vi "Finding-g.vi"() -> ()   [LabVIEW 2021]
uses:
  <userlib>/ImageProcessing/IdentifyBlob_Circle_Cluster.vi
  _SubVis/Ramp.vi
  _SubVis/Bounce.vi
panel:
  out "Cropped Data":dbl[](graph)
  out "Image 3":picture
  in  "stop":bool
  in  "Bounce":bool
  in  "Ramp":bool
  out "Acceleration due to gravity =":dbl
  out "Distance Chart":dbl[](graph)
  # "m/s/s"
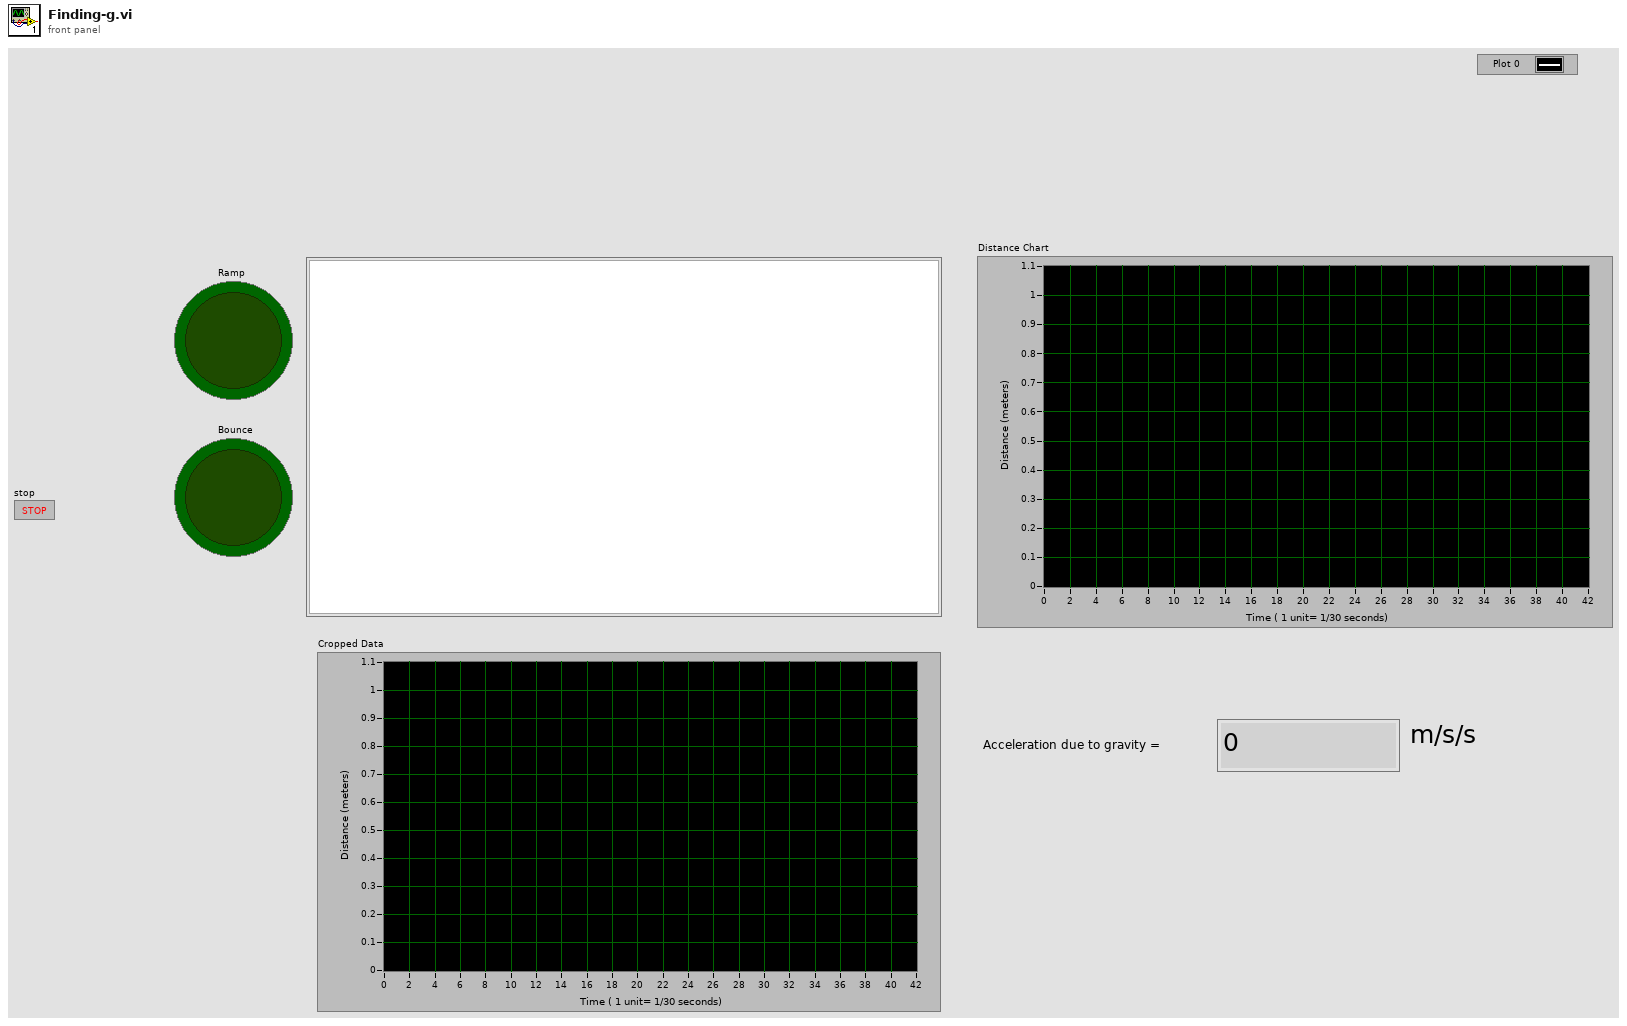
[diagram p1: front panel]
types:
  T1 = typedef "QT_Image.ctl" = cluster{"Width":i32, "Height":i32, "Depth":i32, "data":u8[], "Compressed data":u8[], "Color table":u32[], "Duration":i32, "Options":i32, "Timestamp":i32, "ID":i32, "Reserved":i32, "Dialogs":u32}
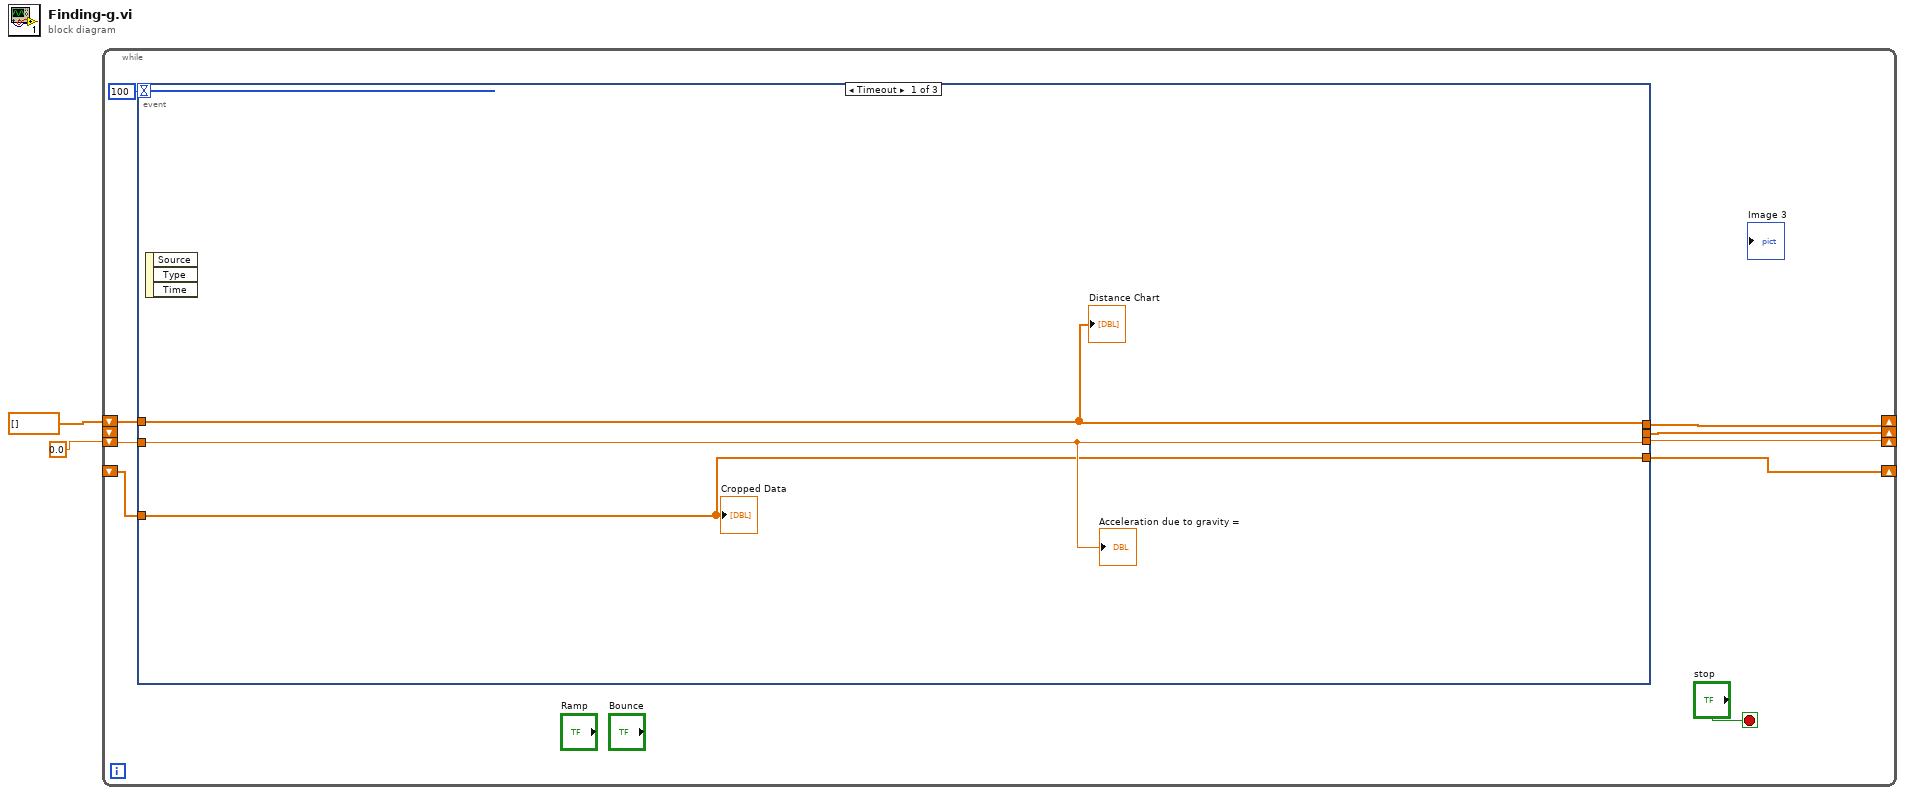
[diagram p0: block diagram]
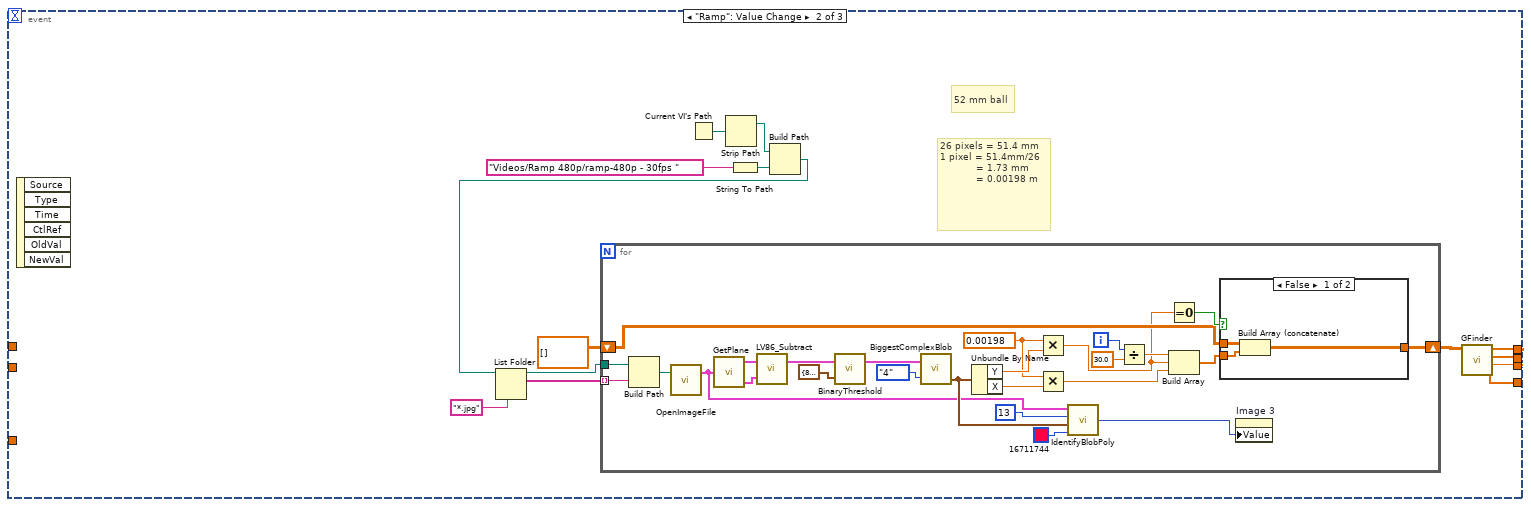
[diagram p2: hidden frame]
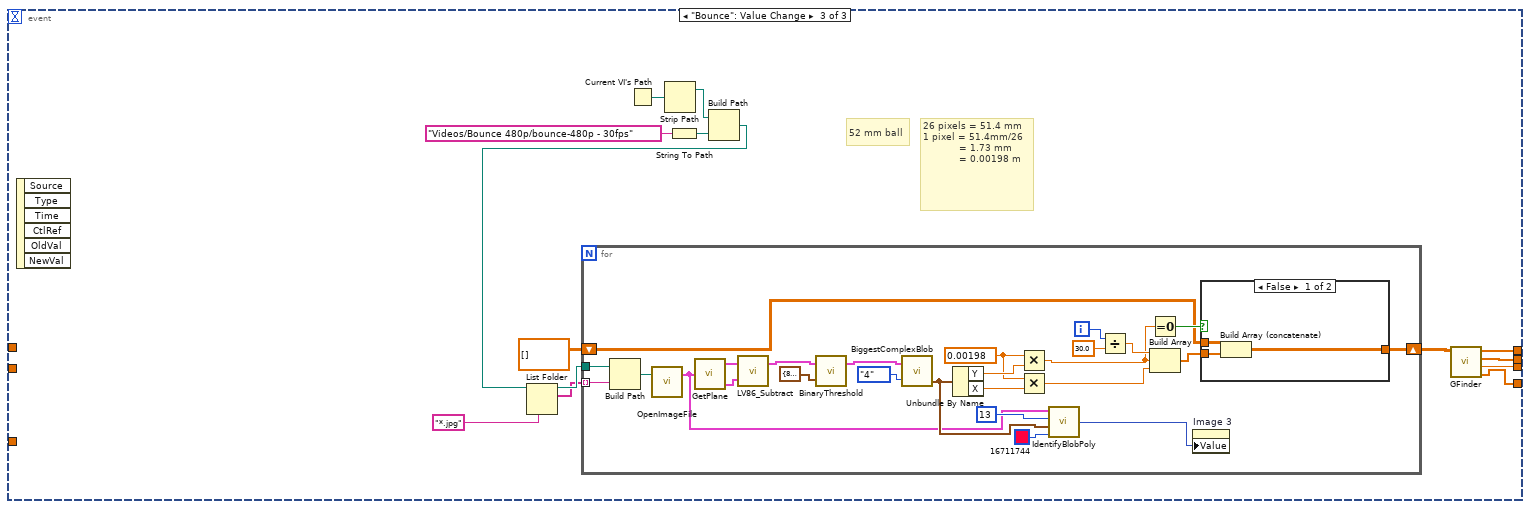
[diagram p4: hidden frame]
diagram:
  n1 = while {
    shift-right: [w7] -> _
    shift-left: dbl[] [] ("Distance") -> [w9]
    shift-right: [w6] -> _
    shift-left: 0.0 ("Acceleration") -> [w8]
    shift-right: [w5] -> _
    shift-left: _ -> [w3]
    shift-right: [w4] -> _
    shift-left: _ -> [_]
    stop <- "stop" stop-if-true
    n2 = event shown="[0] Timeout" {
      selector: _ -> [_ _ _]
      dyn-events: _ -> [_ _ _]
      timeout: 100 -> [_ _ _]
      tunnel: [w14 w22 w71] -> w6
      tunnel: [w13 w23 w72] -> w7
      tunnel: w9 -> [w13 _ _]
      tunnel: w8 -> [w14 _ _]
      tunnel: [w12 w21 w65] -> w5
      tunnel: [_ w20 w64] -> w4
      tunnel: w3 -> [w12 _ _]
      event Timeout {
        n3 = event-data() -> ()  [unwired: 1 in, 3 out]
        "Distance Chart" <- w13
        "Acceleration due to gravity =" <- w14
        "Cropped Data" <- w12
      }
      event "Ramp": Value Change {
        # "26 pixels = 51.4 mm\n1 pixel = 51.4mm/26\n            = 1.73 mm\n            = 0.00198 m"
        # "52 mm ball"
        n4 = event-data() -> ()  [unwired: 1 in, 6 out]
        n5 = Current VI's Path() -> (path=w19:path)
        n6 = Strip Path(path=w19) -> (stripped path=w18:path)  [unwired: 1 out]
        n7 = String To Path(string="Videos/Ramp 480p/ramp-480p - 30fps ") -> (path=w16:path)
        n8 = Build Path(base path=w18, name or relative path=w16) -> (appended path=w15:path)
        n9 = List Folder(path=w15, pattern="*.jpg" ("string")) -> (path out=w27:path, filenames=w26:string[])  [unwired: 2 in, 2 out]
        n10 = for {
          tunnel: w26 -> [w53] mode=indexing
          tunnel: w27 -> [w54]
          shift-right: [w44] -> w24
          shift-left: dbl[][] [] -> [w46]
          i -> [w42]
          w34 = 0.00198 ("x")
          n11 = Build Path(base path=w54, name or relative path=w53) -> (appended path=w52:path)
          n12 = call <userlib>:"OpenImageFile.vi"("selected path"=w52) -> ("Image Out"=w40:T1)  [unwired: 2 in]
          n13 = call <userlib>:"GetPlane.vi"("Image In"=w40) -> ("Blue Plane Out"=w39:T1, "Red Plane Out"=w38:T1)  [unwired: 1 out]
          n14 = call <userlib>:"LV86_Subtract.vi"("Image 2"=w39, "Image"=w38) -> ("Image Out"=w37:T1)  [unwired: 1 in]
          n15 = call <userlib>:"BinaryThreshold.vi"("threshold"=cluster{u8, u8} {82, 120} ("Red Threshold"), "Image In"=w37) -> ("Image Out"=w36:T1)  [unwired: 1 in]
          n16 = call <userlib>:"BiggestComplexBlob.vi"("Connectivity"=enum16{"4", "8"}."4", "Image in"=w36) -> ("Centroid"=w51:cluster{"X":dbl, "Y":dbl})  [unwired: 2 out]
          n17 = Unbundle By Name(w51) -> ("Y"=w48:dbl, "X"=w33:dbl)
          n18 = Multiply(x=w34, y=w48) -> (x*y=w30:dbl)
          n19 = Multiply(x=w34, y=w33) -> (x*y=w32:dbl)
          n20 = call-poly <userlib>:"IdentifyBlobPoly.vi"("color"=u32 16711744, "Centroid"=w51, "Dimension"=13, "Image in"=w40) -> ("picture"=w29:picture)
          n21 = Divide(x=w42, y=30.0 ("x")) -> (x/y=w31:dbl)
          n22 = Equal To 0?(x=w30) -> (x = 0?=w47:bool)
          n23 = Build Array(w31, w30, w32) -> (w45:dbl[])
          n24 = case shown="False" w47 {
            tunnel: w46 -> [w57 w58]
            tunnel: w45 -> [w56 _]
            tunnel: [w55 w58] -> w44
            frame False {
              n25 = Build Array (concatenate)(w57, w56) -> (w55:dbl[][])
            }
            frame True {
              # "to remove all 0 centroids"
            }
          }
          n26 = property on="Image 3" class="Pict"("Value"=w29) -> ()  [unwired: 2 in, 2 out]
        }
        n27 = call-poly "GFinder.vi"("Array"=w24) -> ("Result calculated from"=w21:dbl[], "Acceleration"=w22:dbl, "Time"=w20:dbl[], "Distance"=w23:dbl[])  [unwired: 7 in]
      }
      event "Bounce": Value Change {
        # "26 pixels = 51.4 mm\n1 pixel = 51.4mm/26\n            = 1.73 mm\n            = 0.00198 m"
        # "52 mm ball"
        n28 = event-data() -> ()  [unwired: 1 in, 6 out]
        n29 = Current VI's Path() -> (path=w63:path)
        n30 = Strip Path(path=w63) -> (stripped path=w62:path)  [unwired: 1 out]
        n31 = String To Path(string="Videos/Bounce 480p/bounce-480p - 30fps") -> (path=w60:path)
        n32 = Build Path(base path=w62, name or relative path=w60) -> (appended path=w59:path)
        n33 = List Folder(path=w59, pattern="*.jpg" ("string")) -> (path out=w69:path, filenames=w68:string[])  [unwired: 2 in, 2 out]
        n34 = for {
          tunnel: w68 -> [w97] mode=indexing
          tunnel: w69 -> [w98]
          shift-right: [w88] -> w66
          shift-left: dbl[][] [] -> [w90]
          i -> [w86]
          w78 = 0.00198 ("x")
          n35 = Build Path(base path=w98, name or relative path=w97) -> (appended path=w96:path)
          n36 = call <userlib>:"OpenImageFile.vi"("selected path"=w96) -> ("Image Out"=w84:T1)  [unwired: 2 in]
          n37 = call <userlib>:"GetPlane.vi"("Image In"=w84) -> ("Blue Plane Out"=w83:T1, "Red Plane Out"=w82:T1)  [unwired: 1 out]
          n38 = call <userlib>:"LV86_Subtract.vi"("Image 2"=w83, "Image"=w82) -> ("Image Out"=w81:T1)  [unwired: 1 in]
          n39 = call <userlib>:"BinaryThreshold.vi"("threshold"=cluster{u8, u8} {82, 120} ("Red Threshold"), "Image In"=w81) -> ("Image Out"=w80:T1)  [unwired: 1 in]
          n40 = call <userlib>:"BiggestComplexBlob.vi"("Connectivity"=enum16{"4", "8"}."4", "Image in"=w80) -> ("Centroid"=w95:cluster{"X":dbl, "Y":dbl})  [unwired: 2 out]
          n41 = Unbundle By Name(w95) -> ("Y"=w92:dbl, "X"=w77:dbl)
          n42 = Multiply(x=w78, y=w92) -> (x*y=w74:dbl)
          n43 = Multiply(x=w78, y=w77) -> (x*y=w76:dbl)
          n44 = call-poly <userlib>:"IdentifyBlobPoly.vi"("color"=u32 16711744, "Centroid"=w95, "Dimension"=13, "Image in"=w84) -> ("picture"=w73:picture)
          n45 = Divide(x=w86, y=30.0 ("x")) -> (x/y=w75:dbl)
          n46 = Equal To 0?(x=w74) -> (x = 0?=w91:bool)
          n47 = Build Array(w75, w74, w76) -> (w89:dbl[])
          n48 = property on="Image 3" class="Pict"("Value"=w73) -> ()  [unwired: 2 in, 2 out]
          n49 = case shown="False" w91 {
            tunnel: w90 -> [w101 w102]
            tunnel: w89 -> [w100 _]
            tunnel: [w99 w102] -> w88
            frame False {
              n50 = Build Array (concatenate)(w101, w100) -> (w99:dbl[][])
            }
            frame True {
              # "to remove all 0 centroids"
            }
          }
        }
        n51 = call-poly "GFinder.vi"("Array"=w66) -> ("Result calculated from"=w65:dbl[], "Acceleration"=w71:dbl, "Time"=w64:dbl[], "Distance"=w72:dbl[])  [unwired: 7 in]
      }
    }
  }
